vi "incarcare_harta+pattern_recognition.vi"(10 "Find":path, 11 "Image 2":T1(plugin-control)) -> (3 "Matches (pixel)":T2(array[cluster]))   [LabVIEW 2015]
panel:
  out "Found at":i32
  in  "Minim Matching Points":i32
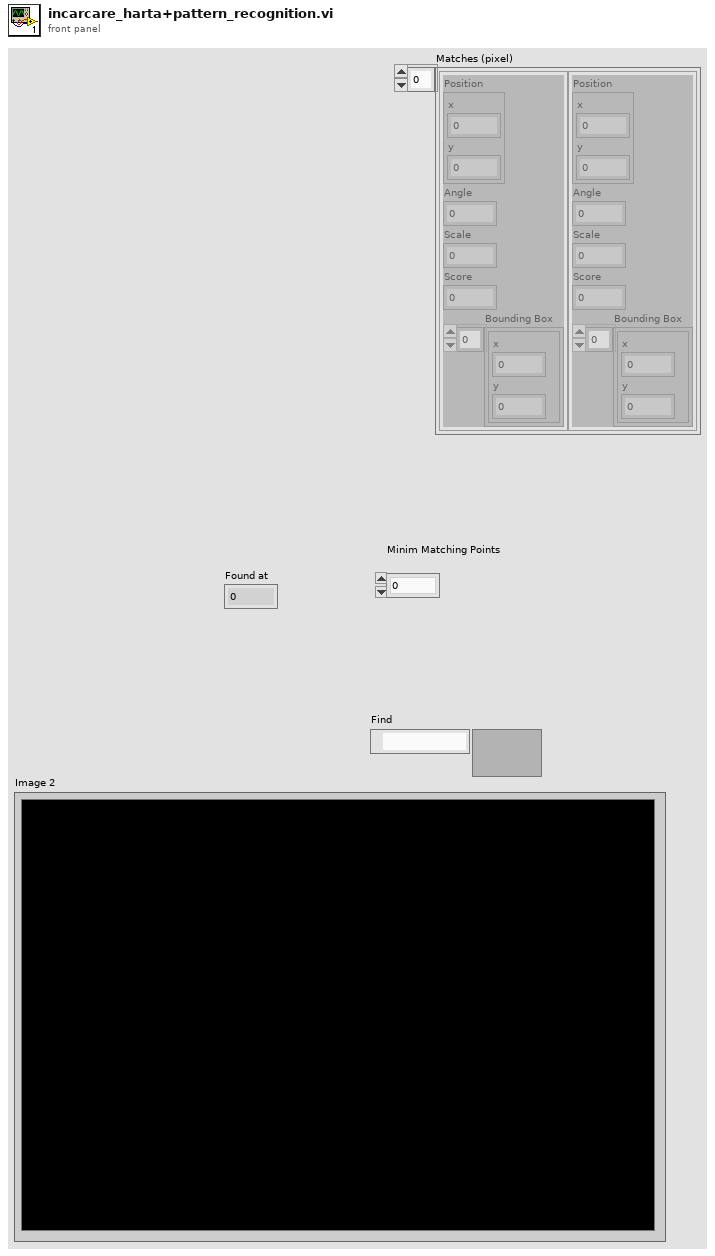
[diagram p1: front panel]
types:
  T1 = typedef "IMAQ Image.ctl" = refnum<image>
  T2 = cluster{"Position":cluster{"x":sgl, "y":sgl}, "Angle":sgl, "Scale":sgl, "Score":sgl, "Bounding Box":cluster{"x":sgl, "y":sgl}[]}[]
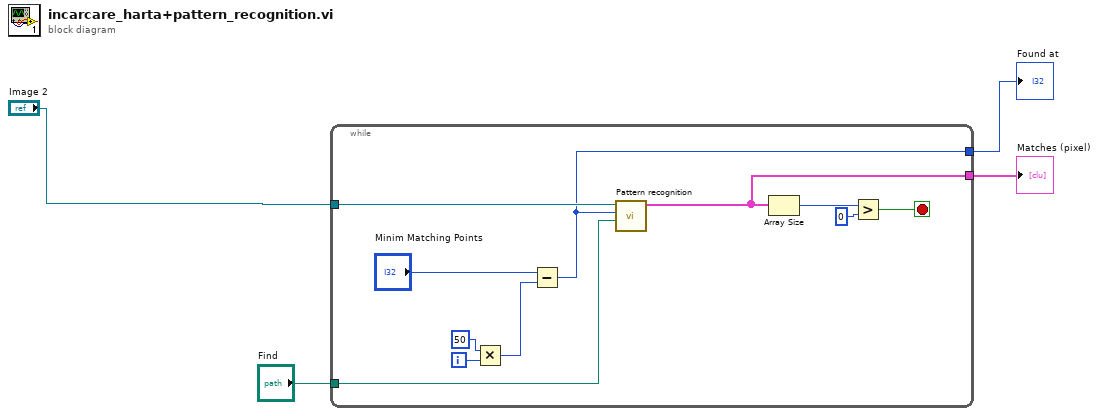
[diagram p0: block diagram]
diagram:
  n1 = while {
    tunnel: "Image 2" -> [w9]
    tunnel: [w8] -> w2
    tunnel: "Find" -> [w6]
    tunnel: [w5] -> w3
    i -> [w12]
    stop <- w7 stop-if-true
    n2 = Multiply(x=50, y=w12) -> (x*y=w10:i32)
    n3 = Subtract(x="Minim Matching Points", y=w10) -> (x-y=w5:i32)
    n4 = call "Pattern recognition.vi"("Template Path"=w6, "Minimum match points"=w5, "Image 2"=w9) -> ("Matches (pixel)"=w8:T2)  [unwired: 8 in]
    n5 = Array Size(array=w8) -> (size(s)=w15:i32)
    n6 = Greater?(x=w15, y=0) -> (0:w7:bool)
  }
  "Found at" <- w3
  "Matches (pixel)" <- w2
